vi "edittest read sequence from file.vi"(8 "error in (no error)":errorcluster, 11 "File Refnum In":T1) -> (0 "error out":errorcluster, 1 "Version":string, 2 "Sequence Record":T2, 3 "File Refnum Out":T1)   [LabVIEW 2011]
uses:
  <vilib>/Utility/config.llb/Config Data RefNum.ctl
  server/database/Sequences/Sequence Record.ctl
  <vilib>/Utility/config.llb/Read Key (String).vi
  <vilib>/Utility/config.llb/Read Key (Double).vi
  <vilib>/Utility/config.llb/Read Key (I32).vi
  <vilib>/Utility/config.llb/Read Key (Boolean).vi
  <vilib>/Utility/config.llb/NI_LVConfig.lvlib
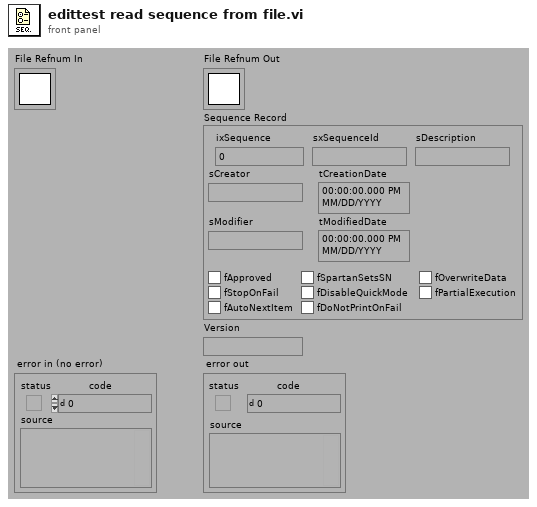
[diagram p1: front panel]
types:
  T1 = typedef "NI_LVConfig.lvlib/Config Data RefNum.ctl" = refnum<k1>
  T2 = typedef "Sequence Record.ctl" = cluster{"ixSequence":i32, "sxSequenceId":string, "sDescription":string, "sCreator":string, "tCreationDate":timestamp, "sModifier":string, "tModifiedDate":timestamp, "fApproved":bool, "fSpartanSetsSN":bool, "fOverwriteData":bool, "fStopOnFail":bool, "fDisableQuickMode":bool, "fPartialExecution":bool, "fAutoNextItem":bool, "fDoNotPrintOnFail":bool}
  T3 = cluster{"Boolean array[0]":bool, "Boolean array[1]":bool}
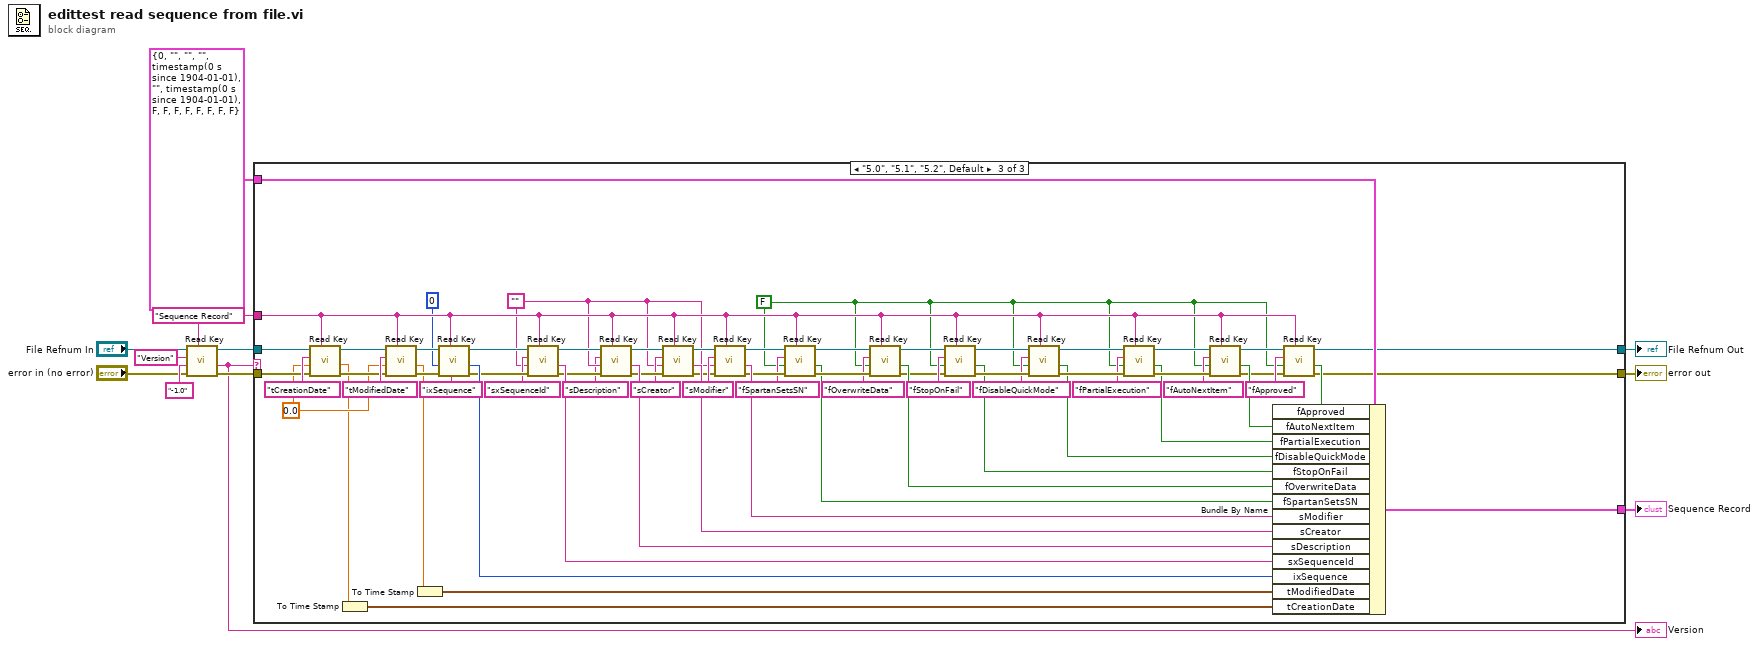
[diagram p0: block diagram]
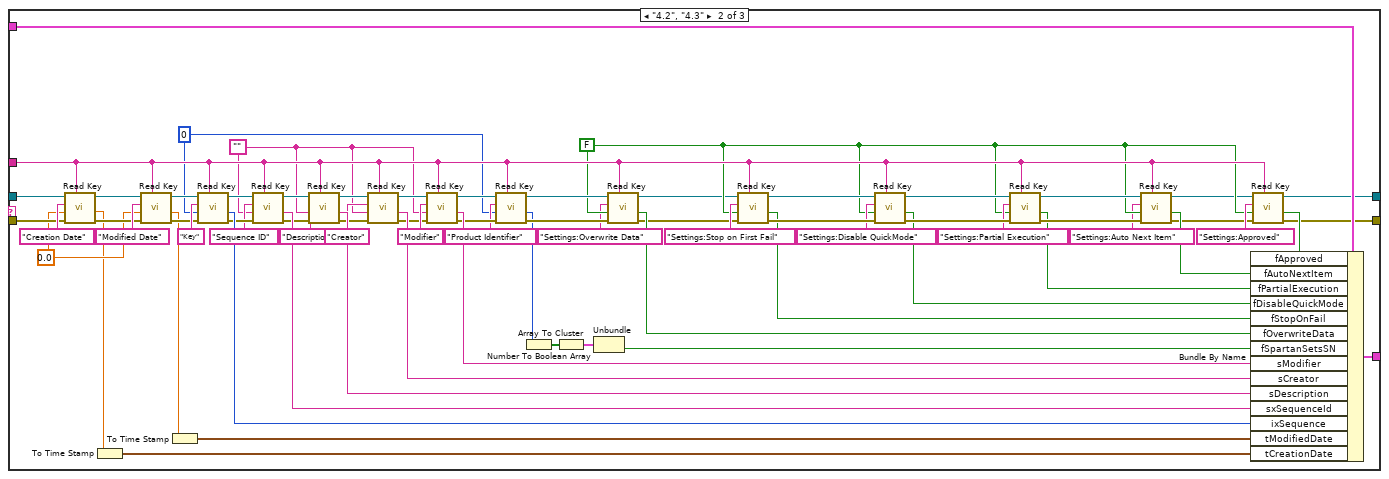
[diagram p3: hidden frame]
diagram:
  w5 = "Sequence Record" ("format string")
  n1 = call-poly <vilib>:"Read Key.vi"("section"=w5, "error in (no error)"="error in (no error)", "default value"="-1.0" ("key"), "key"="Version", "refnum"="File Refnum In") -> ("error out"=w12:errorcluster, "value"=w8:string, "refnum out"=w11:T1)  [unwired: 1 in, 3 out]
  "Version" <- w8
  n2 = case shown="\"5.0\", \"5.1\", \"5.2\", Default" w8 {
    tunnel: [w14 w24 w89] -> w4
    tunnel: [w13 w25 w90] -> w3
    tunnel: w12 -> [w14 w44 w111]
    tunnel: w11 -> [w13 w49 w116]
    tunnel: w5 -> [_ w38 w105]
    tunnel: [_ w37 w104] -> w2
    tunnel: T2 {"ixSequence"=0, "sxSequenceId"="", "sDescription"="", "sCreator"="", "tCreationDate"=timestamp(0 s since 1904-01-01), "sModifier"="", "tModifiedDate"=timestamp(0 s since 1904-01-01), "fApproved"=FALSE, "fSpartanSetsSN"=FALSE, "fOverwriteData"=FALSE, "fStopOnFail"=FALSE, "fDisableQuickMode"=FALSE, "fPartialExecution"=FALSE, "fAutoNextItem"=FALSE, "fDoNotPrintOnFail"=FALSE} ("Sequence Record") -> [_ w36 w103]
    frame "-1.0" {
    }
    frame "4.2", "4.3" {
      w43 = 0.0
      w19 = 0
      w26 = ""
      w34 = FALSE
      n3 = call-poly <vilib>:"Read Key.vi"("section"=w38, "error in (no error)"=w44, "default value"=w43, "key"="Creation Date", "refnum"=w49) -> ("error out"=w45:errorcluster, "value"=w41:dbl, "refnum out"=w48:T1)  [unwired: 4 out]
      n4 = To Time Stamp(1:w41) -> (0:w39:timestamp)
      n5 = call-poly <vilib>:"Read Key.vi"("section"=w38, "error in (no error)"=w45, "default value"=w43, "key"="Modified Date", "refnum"=w48) -> ("error out"=w46:errorcluster, "value"=w42:dbl, "refnum out"=w47:T1)  [unwired: 4 out]
      n6 = To Time Stamp(1:w42) -> (0:w40:timestamp)
      n7 = call-poly <vilib>:"Read Key.vi"("section"=w38, "error in (no error)"=w46, "default value"=w19, "key"="Key", "refnum"=w47) -> ("error out"=w60:errorcluster, "value"=w73:i32, "refnum out"=w67:T1)  [unwired: 4 out]
      n8 = call-poly <vilib>:"Read Key.vi"("section"=w38, "error in (no error)"=w60, "default value"=w26, "key"="Sequence ID", "refnum"=w67) -> ("error out"=w61:errorcluster, "value"=w74:string, "refnum out"=w66:T1)  [unwired: 1 in, 3 out]
      n9 = call-poly <vilib>:"Read Key.vi"("section"=w38, "error in (no error)"=w61, "default value"=w26, "key"="Description", "refnum"=w66) -> ("error out"=w72:errorcluster, "value"=w75:string, "refnum out"=w71:T1)  [unwired: 1 in, 3 out]
      n10 = call-poly <vilib>:"Read Key.vi"("section"=w38, "error in (no error)"=w72, "default value"=w26, "key"="Creator", "refnum"=w71) -> ("error out"=w69:errorcluster, "value"=w76:string, "refnum out"=w70:T1)  [unwired: 1 in, 3 out]
      n11 = call-poly <vilib>:"Read Key.vi"("section"=w38, "error in (no error)"=w69, "default value"=w26, "key"="Modifier", "refnum"=w70) -> ("error out"=w62:errorcluster, "value"=w77:string, "refnum out"=w65:T1)  [unwired: 1 in, 3 out]
      n12 = call-poly <vilib>:"Read Key.vi"("section"=w38, "error in (no error)"=w62, "default value"=w19, "key"="Product Identifier", "refnum"=w65) -> ("error out"=w63:errorcluster, "value"=w16:i32, "refnum out"=w64:T1)  [unwired: 4 out]
      n13 = Number To Boolean Array(number=w16) -> (Boolean array=w18:bool[])
      n14 = Array To Cluster(array=w18) -> (cluster=w17:T3)
      n15 = Unbundle(w17) -> ("Boolean array[1]"=w15:bool)  [unwired: 1 out]
      n16 = call-poly <vilib>:"Read Key.vi"("section"=w38, "error in (no error)"=w63, "default value"=w34, "key"="Settings:Overwrite Data", "refnum"=w64) -> ("error out"=w21:errorcluster, "value"=w35:bool, "refnum out"=w20:T1)  [unwired: 4 out]
      n17 = call-poly <vilib>:"Read Key.vi"("section"=w38, "error in (no error)"=w21, "default value"=w34, "key"="Settings:Stop on First Fail", "refnum"=w20) -> ("error out"=w78:errorcluster, "value"=w33:bool, "refnum out"=w83:T1)  [unwired: 4 out]
      n18 = call-poly <vilib>:"Read Key.vi"("section"=w38, "error in (no error)"=w78, "default value"=w34, "key"="Settings:Disable QuickMode", "refnum"=w83) -> ("error out"=w79:errorcluster, "value"=w32:bool, "refnum out"=w82:T1)  [unwired: 4 out]
      n19 = call-poly <vilib>:"Read Key.vi"("section"=w38, "error in (no error)"=w79, "default value"=w34, "key"="Settings:Partial Execution", "refnum"=w82) -> ("error out"=w80:errorcluster, "value"=w31:bool, "refnum out"=w81:T1)  [unwired: 4 out]
      n20 = call-poly <vilib>:"Read Key.vi"("section"=w38, "error in (no error)"=w80, "default value"=w34, "key"="Settings:Auto Next Item", "refnum"=w81) -> ("error out"=w23:errorcluster, "value"=w30:bool, "refnum out"=w22:T1)  [unwired: 4 out]
      n21 = call-poly <vilib>:"Read Key.vi"("section"=w38, "error in (no error)"=w23, "default value"=w34, "key"="Settings:Approved", "refnum"=w22) -> ("error out"=w24:errorcluster, "value"=w29:bool, "refnum out"=w25:T1)  [unwired: 4 out]
      n22 = Bundle By Name(cluster=w36, "fApproved"=w29, "fAutoNextItem"=w30, "fPartialExecution"=w31, "fDisableQuickMode"=w32, "fStopOnFail"=w33, "fOverwriteData"=w35, "fSpartanSetsSN"=w15, "sModifier"=w77, "sCreator"=w76, "sDescription"=w75, "sxSequenceId"=w74, "ixSequence"=w73, "tModifiedDate"=w40, "tCreationDate"=w39) -> (w37:T2)
    }
    frame "5.0", "5.1", "5.2", Default {
      w110 = 0.0
      w86 = ""
      w88 = FALSE
      n23 = call-poly <vilib>:"Read Key.vi"("section"=w105, "error in (no error)"=w111, "default value"=w110, "key"="tCreationDate", "refnum"=w116) -> ("error out"=w112:errorcluster, "value"=w108:dbl, "refnum out"=w115:T1)  [unwired: 4 out]
      n24 = To Time Stamp(1:w108) -> (0:w106:timestamp)
      n25 = call-poly <vilib>:"Read Key.vi"("section"=w105, "error in (no error)"=w112, "default value"=w110, "key"="tModifiedDate", "refnum"=w115) -> ("error out"=w113:errorcluster, "value"=w109:dbl, "refnum out"=w114:T1)  [unwired: 4 out]
      n26 = To Time Stamp(1:w109) -> (0:w107:timestamp)
      n27 = call-poly <vilib>:"Read Key.vi"("section"=w105, "error in (no error)"=w113, "default value"=0, "key"="ixSequence", "refnum"=w114) -> ("error out"=w127:errorcluster, "value"=w140:i32, "refnum out"=w134:T1)  [unwired: 4 out]
      n28 = call-poly <vilib>:"Read Key.vi"("section"=w105, "error in (no error)"=w127, "default value"=w86, "key"="sxSequenceId", "refnum"=w134) -> ("error out"=w128:errorcluster, "value"=w141:string, "refnum out"=w133:T1)  [unwired: 1 in, 3 out]
      n29 = call-poly <vilib>:"Read Key.vi"("section"=w105, "error in (no error)"=w128, "default value"=w86, "key"="sDescription", "refnum"=w133) -> ("error out"=w139:errorcluster, "value"=w142:string, "refnum out"=w138:T1)  [unwired: 1 in, 3 out]
      n30 = call-poly <vilib>:"Read Key.vi"("section"=w105, "error in (no error)"=w139, "default value"=w86, "key"="sCreator", "refnum"=w138) -> ("error out"=w136:errorcluster, "value"=w143:string, "refnum out"=w137:T1)  [unwired: 1 in, 3 out]
      n31 = call-poly <vilib>:"Read Key.vi"("section"=w105, "error in (no error)"=w136, "default value"=w86, "key"="sModifier", "refnum"=w137) -> ("error out"=w129:errorcluster, "value"=w144:string, "refnum out"=w132:T1)  [unwired: 1 in, 3 out]
      n32 = call-poly <vilib>:"Read Key.vi"("section"=w105, "error in (no error)"=w129, "default value"=w88, "key"="fSpartanSetsSN", "refnum"=w132) -> ("error out"=w130:errorcluster, "value"=w124:bool, "refnum out"=w131:T1)  [unwired: 4 out]
      n33 = call-poly <vilib>:"Read Key.vi"("section"=w105, "error in (no error)"=w130, "default value"=w88, "key"="fOverwriteData", "refnum"=w131) -> ("error out"=w94:errorcluster, "value"=w102:bool, "refnum out"=w93:T1)  [unwired: 4 out]
      n34 = call-poly <vilib>:"Read Key.vi"("section"=w105, "error in (no error)"=w94, "default value"=w88, "key"="fStopOnFail", "refnum"=w93) -> ("error out"=w145:errorcluster, "value"=w101:bool, "refnum out"=w150:T1)  [unwired: 4 out]
      n35 = call-poly <vilib>:"Read Key.vi"("section"=w105, "error in (no error)"=w145, "default value"=w88, "key"="fDisableQuickMode", "refnum"=w150) -> ("error out"=w146:errorcluster, "value"=w100:bool, "refnum out"=w149:T1)  [unwired: 4 out]
      n36 = call-poly <vilib>:"Read Key.vi"("section"=w105, "error in (no error)"=w146, "default value"=w88, "key"="fPartialExecution", "refnum"=w149) -> ("error out"=w147:errorcluster, "value"=w99:bool, "refnum out"=w148:T1)  [unwired: 4 out]
      n37 = call-poly <vilib>:"Read Key.vi"("section"=w105, "error in (no error)"=w147, "default value"=w88, "key"="fAutoNextItem", "refnum"=w148) -> ("error out"=w92:errorcluster, "value"=w98:bool, "refnum out"=w91:T1)  [unwired: 4 out]
      n38 = call-poly <vilib>:"Read Key.vi"("section"=w105, "error in (no error)"=w92, "default value"=w88, "key"="fApproved", "refnum"=w91) -> ("error out"=w89:errorcluster, "value"=w97:bool, "refnum out"=w90:T1)  [unwired: 4 out]
      n39 = Bundle By Name(cluster=w103, "fApproved"=w97, "fAutoNextItem"=w98, "fPartialExecution"=w99, "fDisableQuickMode"=w100, "fStopOnFail"=w101, "fOverwriteData"=w102, "fSpartanSetsSN"=w124, "sModifier"=w144, "sCreator"=w143, "sDescription"=w142, "sxSequenceId"=w141, "ixSequence"=w140, "tModifiedDate"=w107, "tCreationDate"=w106) -> (w104:T2)
    }
  }
  "error out" <- w4
  "Sequence Record" <- w2
  "File Refnum Out" <- w3
